vi "StringArray in comma separated String.vi"(11 "Component Names":T1[](array[typedef])) -> (3 "String":string)   [LabVIEW 2020, in "Linearisierung v2.lvlib" / "SpanEinstellungen.lvlib"]
uses:
  SpanEinstellungen.lvlib
  Visualisierungs Elemente/String - Ausgabefeld.ctl
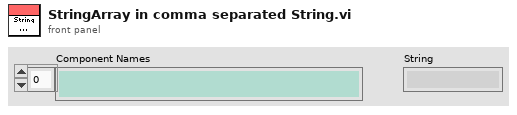
[diagram p1: front panel]
types:
  T1 = typedef "String - Ausgabefeld.ctl" = string
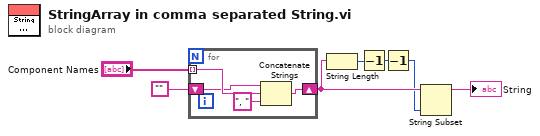
[diagram p0: block diagram]
diagram:
  n1 = for {
    tunnel: "Component Names" -> [w11] mode=indexing
    shift-right: [w10] -> w7
    shift-left: "" -> [w9]
    n2 = Concatenate Strings(w9, w11, T1 ", " ("String")) -> (w10:string)
  }
  n3 = String Length(string=w7) -> (length=w3:i32)
  n4 = Decrement(x=w3) -> (x-1=w2:i32)
  n5 = Decrement(x=w2) -> (x-1=w1:i32)
  n6 = String Subset(string=w7, length (rest)=w1) -> (substring=→"String":string)  [unwired: 1 in]
